vi "Catapulta Disponible Global.vi"() -> ()   [LabVIEW 2015]
panel:
  in  "Can shoot":bool
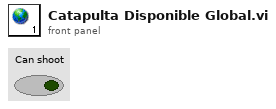
[diagram p1: front panel]
diagram:
